vi "login.vi"() -> (1 "Pass":bool, 2 "Username 2":string, 3 "Password 2":string)   [LabVIEW 2014]
panel:
  in  "enter":bool
  in  "Password":string
  in  "Username":string
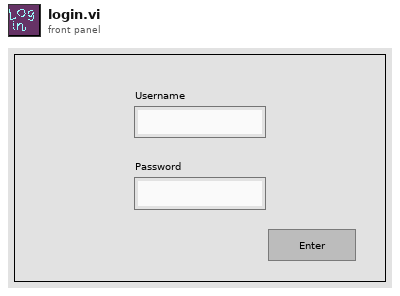
[diagram p1: front panel]
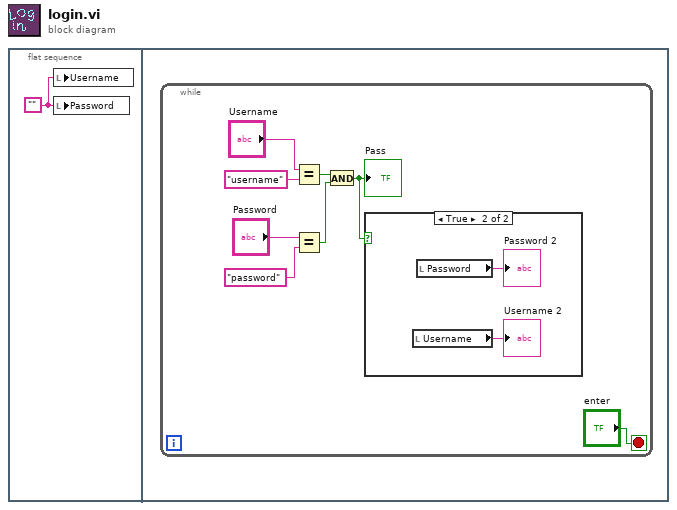
[diagram p0: block diagram]
diagram:
  n1 = flat-sequence {
    frame #0 {
      w1 = ""
      n2 = local write "Username"(w1) -> ()
      n3 = local write "Password"(w1) -> ()
    }
    frame #1 {
      n4 = while {
        stop <- "enter" stop-if-true
        n5 = Equal?(x="Username", y="username") -> (x = y?=w7:bool)
        n6 = Equal?(x="Password", y="password") -> (x = y?=w3:bool)
        n7 = And(x=w7, y=w3) -> (x .and. y?=w2:bool)
        "Pass" <- w2
        n8 = case shown="True" w2 {
          frame False {
          }
          frame True {
            n9 = local read "Username"() -> (→"Username 2":string)
            n10 = local read "Password"() -> (→"Password 2":string)
          }
        }
      }
    }
  }
